vi "飞行姿态模拟.vi"() -> ()   [LabVIEW 8.6]
uses:
  <vilib>/picture/3D Picture Control/NI_3D Picture Control.lvlib
  <vilib>/picture/3D Picture Control/Object/Create Object (name).vi
  <vilib>/picture/3D Picture Control/Object/Add Object (reference).vi
  <vilib>/Utility/miscctls.llb/LVRGBAColorTypeDef.ctl
panel:
  in  "退出按钮":bool
  in  "Yaw":dbl(knob)
  in  "Roll":dbl(knob)
  in  "Pitch":dbl(knob)
  out "三维图片":refnum<vi>(3d-picture)
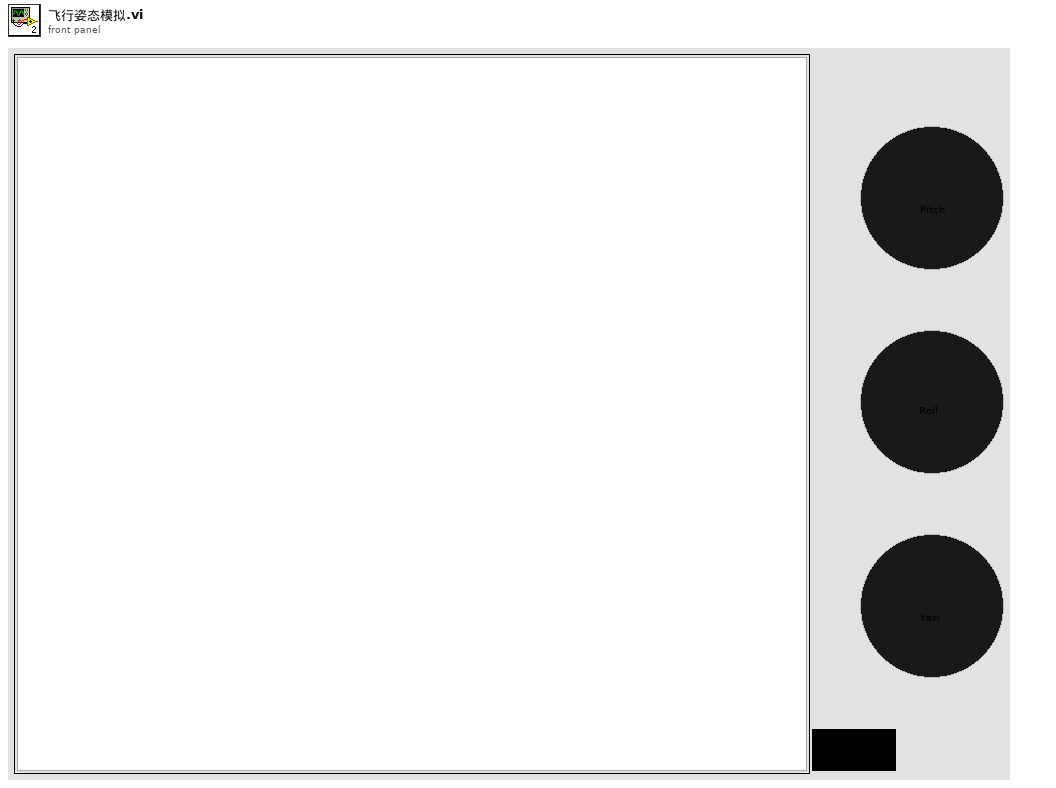
[diagram p1: front panel]
types:
  T1 = typedef "LVRGBAColorTypeDef.ctl" = cluster{"Red":sgl, "Green":sgl, "Blue":sgl, "Alpha":sgl}
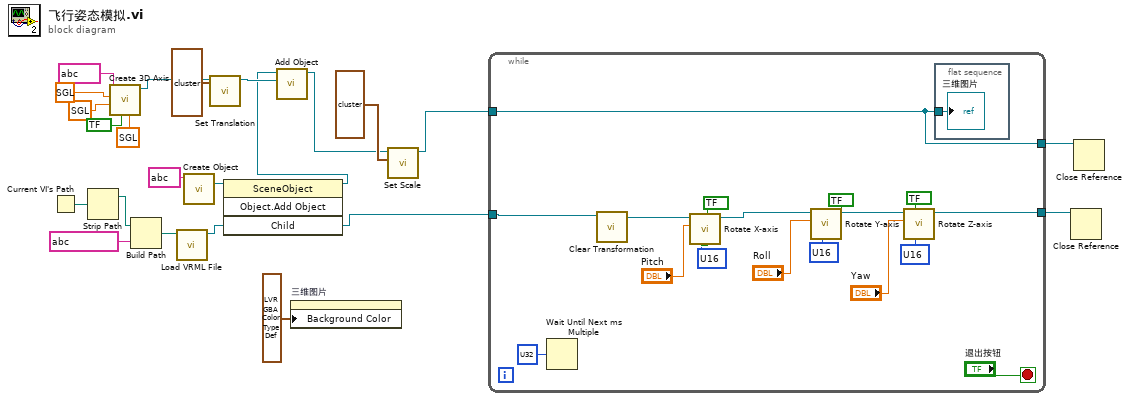
[diagram p0: block diagram]
diagram:
  n1 = Current VI's Path() -> (path=w21:path)
  n2 = Strip Path ("拆分路径")(path=w21) -> (stripped path=w20:path)  [unwired: 1 out]
  n3 = call <vilib>:"Create 3D Axis.vi"("Character Size"=sgl ?, "Axis label?"=bool ?, "Radius"=sgl ?, "Length"=sgl ?, "Name"=string ?) -> ("New Object Refnum"=w6:refnum<vi>)  [unwired: 5 in, 1 out]
  n4 = Build Path ("创建路径")(base path=w20, name or relative path=string ? ("名称或相对路径")) -> (appended path=w18:path)
  n5 = call <vilib>:"Load VRML File.vi"("Path"=w18) -> ("Scene:Read Scene File"=w14:refnum<vi>)  [unwired: 9 in, 1 out]
  n6 = call-poly <vilib>:"Create Object.vi"("Name"=string ?) -> ("Scene:New Object"=w17:refnum<vi>)  [unwired: 9 in, 1 out]
  n7 = call <vilib>:"Set Translation.vi"("Translation"=cluster{"X":sgl, "Y":sgl, "Z":sgl} ?, "Scene Object"=w6) -> ("Translated Object"=w5:refnum<vi>)  [unwired: 8 in, 1 out]
  n8 = invoke class="SceneObject" method="Object.Add Object"(reference=w17, "Child"=w14) -> (reference out=w4:refnum<vi>, "Child"=w3:refnum<vi>)  [unwired: 2 in, 2 out]
  n9 = call-poly <vilib>:"Add Object.vi"("New Object In"=w5, "Scene Object In"=w4) -> ("Scene Object Out"=w7:refnum<vi>)  [unwired: 7 in, 2 out]
  n10 = property on="三维图片" class="SceneGraphDisp (严格)"("Background Color"=T1 ? ("背景色")) -> ()  [unwired: 2 in, 2 out]
  n11 = call <vilib>:"Set Scale.vi"("Scale"=cluster{"X":sgl, "Y":sgl, "Z":sgl} ?, "Scene Object"=w7) -> ("Scaled Object"=w2:refnum<vi>)  [unwired: 8 in, 1 out]
  n12 = while {
    tunnel: w2 -> [w31]
    tunnel: w3 -> [w32]
    tunnel: [w31] -> w23
    tunnel: [w30] -> w22
    stop <- "退出按钮" stop-if-true
    w37 = u16 ? items=["度", "弧度"] ("angle unit")
    w38 = u16 ? items=["度", "弧度"] ("angle unit")
    w39 = u16 ? items=["度", "弧度"] ("angle unit")
    n13 = Wait Until Next ms Multiple(millisecond multiple=u32 ? ("毫秒倍数")) -> ()  [unwired: 1 out]
    n14 = call <vilib>:"Clear Transformation.vi"("Object Refnum In"=w32) -> ("Object Refnum Out"=w34:refnum<vi>)  [unwired: 9 in, 1 out]
    n15 = call <vilib>:"Rotate X-axis.vi"("angle unit"=w39, "Relative?"=bool ?, "angle"="Pitch", "Scene Object In"=w34) -> ("Scene Object Out"=w36:refnum<vi>)  [unwired: 6 in, 1 out]
    n16 = call <vilib>:"Rotate Y-axis.vi"("angle unit"=w38, "Relative?"=bool ?, "angle"="Roll", "Scene Object In"=w36) -> ("Scene Object Out"=w35:refnum<vi>)  [unwired: 6 in, 1 out]
    n17 = call <vilib>:"Rotate Z-axis.vi"("angle unit"=w37, "Relative?"=bool ?, "angle"="Yaw", "Scene Object In"=w35) -> ("Scene Object Out"=w30:refnum<vi>)  [unwired: 6 in, 1 out]
    n18 = flat-sequence {
      tunnel: w31 -> [w41]
      frame #0 {
        "三维图片" <- w41
      }
    }
  }
  n19 = Close Reference(reference=w22) -> ()  [unwired: 1 in, 1 out]
  n20 = Close Reference(reference=w23) -> ()  [unwired: 1 in, 1 out]
